vi "multilistbox.vi"() -> ()   [LabVIEW 2021]
panel:
  in  "Multicolumn Listbox":i32(listbox)
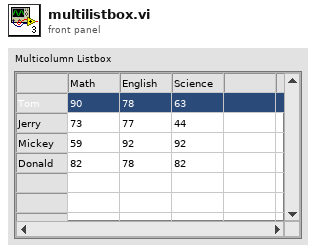
[diagram p1: front panel]
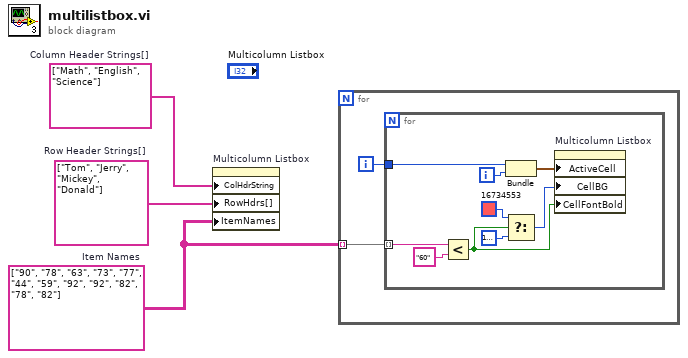
[diagram p0: block diagram]
diagram:
  w2 = string[] ["Tom", "Jerry", "Mickey", "Donald"]  # Row Header Strings[]
  w3 = string[] ["Math", "English", "Science"]  # Column Header Strings[]
  w1 = string[][] [["90", "78", "63"], ["73", "77", "44"], ["59", "92", "92"], ["82", "78", "82"]]  # Item Names
  n1 = property on="Multicolumn Listbox" class="MCListbox (strict)"("ColHdrString"=w3, "RowHdrs[]"=w2, "ItemNames"=w1) -> ()  [unwired: 2 in, 2 out]
  n2 = for {
    tunnel: w1 -> [w5] mode=indexing
    i -> [w4]
    n3 = for {
      tunnel: w5 -> [w14] mode=indexing
      tunnel: w4 -> [w12]
      i -> [w11]
      n4 = Less?(x=w14, y="60") -> (x < y?=w9:bool)
      n5 = Bundle(w12, w11) -> (w10:cluster{i32, i32})  [unwired: 1 in]
      n6 = Select(t=u32 16734553, s=w9, f=u32 16777216) -> (s? t:f=w6:u32)
      n7 = property on="Multicolumn Listbox" class="MCListbox (strict)"("ActiveCell"=w10, "CellBG"=w6, "CellFontBold"=w9) -> ()  [unwired: 2 in, 2 out]
    }
  }
